vi "BufferConfig.vi"(8 "error in (no error)":errorcluster, 9 "Buffer Size [Samps per Chan]":i32=500000, 11 "WaveformTask in":refnum<class "WaveformTask.lvclass">) -> (0 "error out":errorcluster, 1 "Buffer Size [Total Samples]":u32=500000, 3 "WaveformTask out":refnum<class "WaveformTask.lvclass">)   [LabVIEW 2015, in "WaveformTask.lvclass"]
uses:
  WaveformTask.lvclass
  WaveformTask.lvclass/WaveformTask.ctl
  <vilib>/Utility/error.llb/Error Cluster From Error Code.vi
  <vilib>/rvi/interface/common/niFpgaWaitOnOcc.vi
  DataFIFOs.ctl
  <vilib>/rvi/interface/nirviMethod/nirviMethod.xnode
  <vilib>/rvi/errors/niLvFpgaMergeErrorWithErrorCode.vi
  <vilib>/FPGAPlugInAG/Dynamic/niLvFpga_ConfigureFifo_Dynamic.vi
  <vilib>/FPGAPlugInAG/Dynamic/niLvFpga_StartFifo_Dynamic.vi
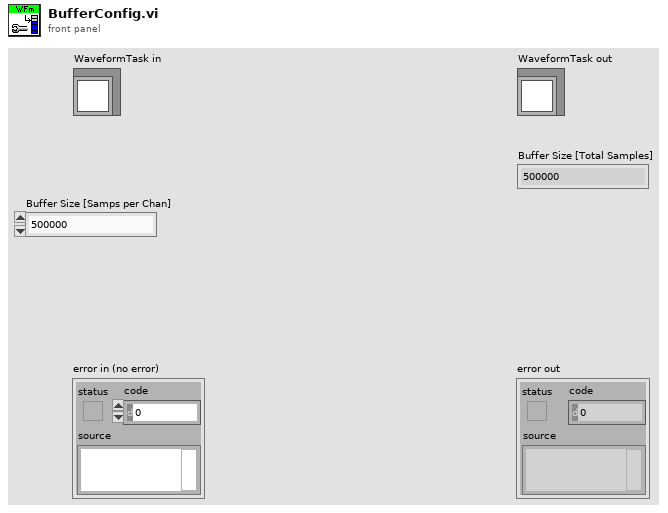
[diagram p1: front panel]
types:
  T1 = typedef "WaveformTask.lvclass/DataFIFOs.ctl" = refnum<k20>
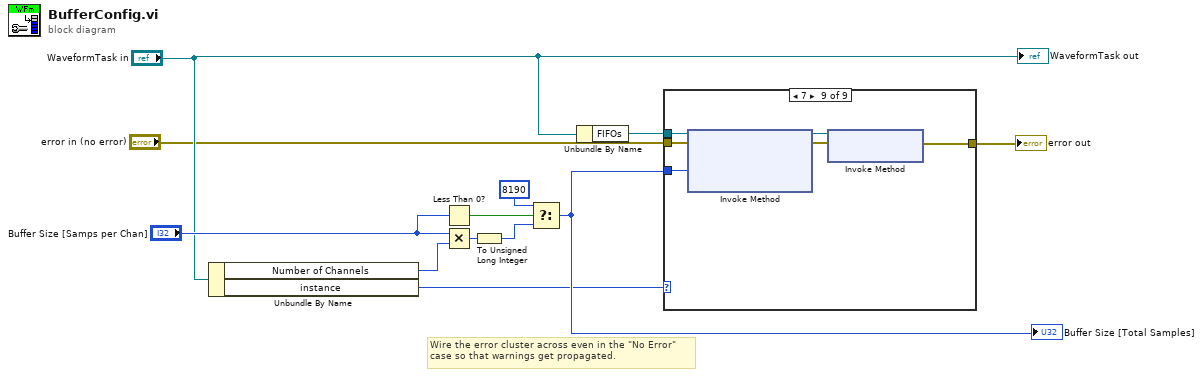
[diagram p0: block diagram]
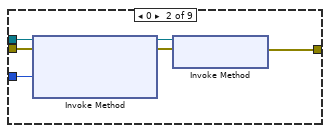
[diagram p3: hidden frame]
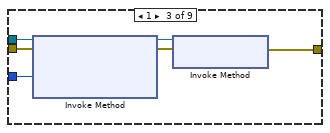
[diagram p4: hidden frame]
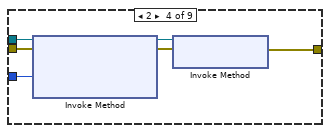
[diagram p5: hidden frame]
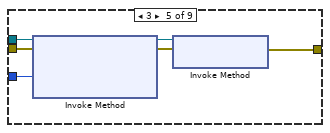
[diagram p6: hidden frame]
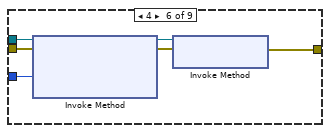
[diagram p7: hidden frame]
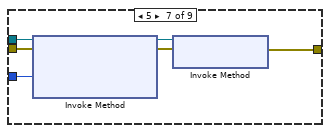
[diagram p8: hidden frame]
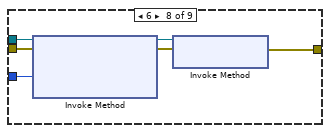
[diagram p9: hidden frame]
diagram:
  # "Wire the error cluster across even in the \"No Error\"\ncase so that warnings get propagated."
  n1 = Unbundle By Name("WaveformTask in") -> ("Number of Channels"=w12:i32, "instance"=w1:u8)
  n2 = Less Than 0?(x="Buffer Size [Samps per Chan]") -> (x < 0?=w7:bool)
  n3 = Multiply(x="Buffer Size [Samps per Chan]", y=w12) -> (x*y=w11:i32)
  n4 = To Unsigned Long Integer(number=w11) -> (unsigned 32bit integer=w10:u32)
  n5 = Select(t=u32 8190 ("unsigned 32bit integer"), s=w7, f=w10) -> (s? t:f=w4:u32)
  "Buffer Size [Total Samples]" <- w4
  n6 = Unbundle By Name("WaveformTask in") -> ("FIFOs"=w5:T1)
  n7 = case shown="7" w1 {
    tunnel: w5 -> [_ w17 w23 w29 w35 w41 w47 w53 w59]
    tunnel: w4 -> [_ w16 w22 w28 w34 w40 w46 w52 w58]
    tunnel: "error in (no error)" -> [w13 w15 w21 w27 w33 w39 w45 w51 w57]
    tunnel: [w13 w14 w20 w26 w32 w38 w44 w50 w56] -> w2
    frame Default {
      # "#TODO error"
    }
    frame 0 {
      n8 = xnode "Invoke Method"("FPGA VI Reference In"=w17, "error in"=w15, "Requested Depth"=w16) -> ("FPGA VI Reference Out"=w19:T1, "error out"=w18:errorcluster)  [unwired: 1 out]
      n9 = xnode "Invoke Method"("FPGA VI Reference In"=w19, "error in"=w18) -> ("error out"=w14:errorcluster)  [unwired: 1 out]
    }
    frame 1 {
      n10 = xnode "Invoke Method"("FPGA VI Reference In"=w23, "error in"=w21, "Requested Depth"=w22) -> ("FPGA VI Reference Out"=w25:T1, "error out"=w24:errorcluster)  [unwired: 1 out]
      n11 = xnode "Invoke Method"("FPGA VI Reference In"=w25, "error in"=w24) -> ("error out"=w20:errorcluster)  [unwired: 1 out]
    }
    frame 2 {
      n12 = xnode "Invoke Method"("FPGA VI Reference In"=w29, "error in"=w27, "Requested Depth"=w28) -> ("FPGA VI Reference Out"=w31:T1, "error out"=w30:errorcluster)  [unwired: 1 out]
      n13 = xnode "Invoke Method"("FPGA VI Reference In"=w31, "error in"=w30) -> ("error out"=w26:errorcluster)  [unwired: 1 out]
    }
    frame 3 {
      n14 = xnode "Invoke Method"("FPGA VI Reference In"=w35, "error in"=w33, "Requested Depth"=w34) -> ("FPGA VI Reference Out"=w37:T1, "error out"=w36:errorcluster)  [unwired: 1 out]
      n15 = xnode "Invoke Method"("FPGA VI Reference In"=w37, "error in"=w36) -> ("error out"=w32:errorcluster)  [unwired: 1 out]
    }
    frame 4 {
      n16 = xnode "Invoke Method"("FPGA VI Reference In"=w41, "error in"=w39, "Requested Depth"=w40) -> ("FPGA VI Reference Out"=w43:T1, "error out"=w42:errorcluster)  [unwired: 1 out]
      n17 = xnode "Invoke Method"("FPGA VI Reference In"=w43, "error in"=w42) -> ("error out"=w38:errorcluster)  [unwired: 1 out]
    }
    frame 5 {
      n18 = xnode "Invoke Method"("FPGA VI Reference In"=w47, "error in"=w45, "Requested Depth"=w46) -> ("FPGA VI Reference Out"=w49:T1, "error out"=w48:errorcluster)  [unwired: 1 out]
      n19 = xnode "Invoke Method"("FPGA VI Reference In"=w49, "error in"=w48) -> ("error out"=w44:errorcluster)  [unwired: 1 out]
    }
    frame 6 {
      n20 = xnode "Invoke Method"("FPGA VI Reference In"=w53, "error in"=w51, "Requested Depth"=w52) -> ("FPGA VI Reference Out"=w55:T1, "error out"=w54:errorcluster)  [unwired: 1 out]
      n21 = xnode "Invoke Method"("FPGA VI Reference In"=w55, "error in"=w54) -> ("error out"=w50:errorcluster)  [unwired: 1 out]
    }
    frame 7 {
      n22 = xnode "Invoke Method"("FPGA VI Reference In"=w59, "error in"=w57, "Requested Depth"=w58) -> ("FPGA VI Reference Out"=w61:T1, "error out"=w60:errorcluster)  [unwired: 1 out]
      n23 = xnode "Invoke Method"("FPGA VI Reference In"=w61, "error in"=w60) -> ("error out"=w56:errorcluster)  [unwired: 1 out]
    }
  }
  "error out" <- w2
  "WaveformTask out" <- "WaveformTask in"
